vi "Untitled 1.vi"   [LabVIEW 2012]
types:
  T1 = enum16{"open", "replace", "create", "open or create", "replace or create", "replace or create with confirmation"}
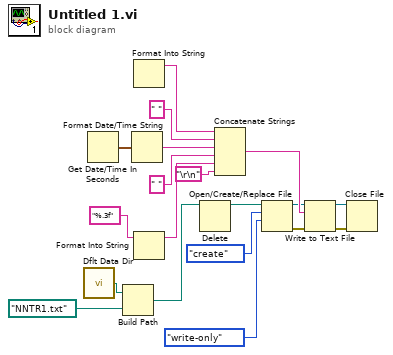
[diagram p0: block diagram]
diagram:
  n1 = call <vilib>:"Dflt Data Dir.vi"() -> ("App:Default Data Directory"=w18:path)
  n2 = Get Date/Time In Seconds() -> (seconds since 1Jan1904=w11:timestamp)
  n3 = Build Path(base path=w18, name or relative path=path "NNTR1.txt" ("Path")) -> (appended path=w17:path)
  n4 = Format Date/Time String(seconds (now)=w11) -> (date/time string=w13:string)  [unwired: 2 in]
  n5 = Format Into String() -> (resulting string=w10:string)  [unwired: 4 in, 1 out]
  n6 = Format Into String(format string="%.3f") -> (resulting string=w12:string)  [unwired: 3 in, 1 out]
  n7 = Delete(path (use dialog)=w17) -> (deleted path=w16:path)  [unwired: 4 in, 2 out]
  n8 = Concatenate Strings(w10, " " ("string"), w13, " " ("string"), w12, "\r\n") -> (w9:string)
  n9 = Open/Create/Replace File(file path (use dialog)=w16, operation (0:open)=T1."create", access (0:read/write)=enum16{"read/write", "read-only", "write-only"}."write-only") -> (refnum out=w3:refnum<file>, error out=w4:errorcluster)  [unwired: 3 in, 1 out]
  n10 = Write to Text File(file (use dialog)=w3, text=w9, error in=w4) -> (refnum out=w1:refnum<file>, error out=w2:errorcluster)  [unwired: 1 in, 1 out]
  n11 = Close File(refnum=w1, error in=w2) -> ()  [unwired: 2 out]
